vi "Exchange State.vi"(8 "error in (no error)":errorcluster, 9 "Throttle":sgl, 10 "Steering":sgl, 11 "FormulaG API in":refnum<class "FormulaG API.lvclass">) -> (0 "error out":errorcluster, 1 "Paused":bool, 2 "Car State":T1 {"Last Lap" format="%<%M:%S%3u>t"; "Current Lap" format="%<%M:%S%3u>t"}, 3 "FormulaG API out":refnum<class "FormulaG API.lvclass">)   [LabVIEW 2024, in "FormulaG.lvlib" / "FormulaG API.lvclass"]
uses:
  FormulaG API.lvclass
  FormulaG-Common/Car State.ctl
  FormulaG-Common/Ranges.ctl
  FormulaG-Common/Car Info.ctl
  Command.ctl
  FormulaG-Common/Car Control.ctl
  FormulaG API.lvclass/FormulaG API.ctl
  FormulaG-Common/FormulaG-Common.lvlib
  <vilib>/IlluminatedG/IG GodotServer/GodotLV/GodotServer/GodotServer.lvclass
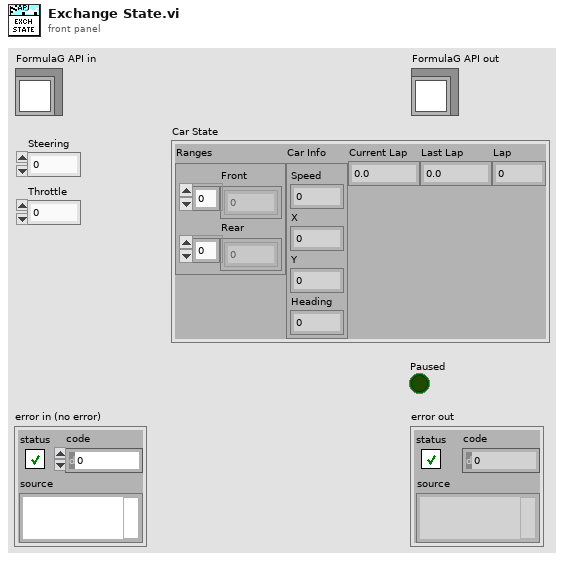
[diagram p1: front panel]
types:
  T1 = typedef "FormulaG-Common.lvlib/Car State.ctl" = cluster{"Ranges":T2, "Car Info":T3, "Current Lap":dbl, "Last Lap":dbl, "Lap":u8}
  T2 = typedef "FormulaG-Common.lvlib/Ranges.ctl" = cluster{"Front":sgl[], "Rear":sgl[]}
  T3 = typedef "FormulaG-Common.lvlib/Car Info.ctl" = cluster{"Speed":sgl, "X":sgl, "Y":sgl, "Heading":sgl}
  T4 = enum16{"big-endian, network order", "native, host order", "little-endian"}
  T5 = typedef "FormulaG-Common.lvlib/Car Control.ctl" = cluster{"Steering (-1 to 1)":sgl, "Throttle (0 to 1)":sgl}
  T6 = cluster{"ID":u8, "Ranges":sgl[], "Info":T3, "Current Lap mS":i64, "Last Lap mS":i64, "Lap":u8, "Paused":u8}
  T7 = typedef "FormulaG.lvlib/FormulaG API.lvclass/Command.ctl" = enum8{"None", "Reset Car", "Request State", "Control Car", "Request Info", "Set Options", "Set Camera", "Set Pause", "Request Time"}
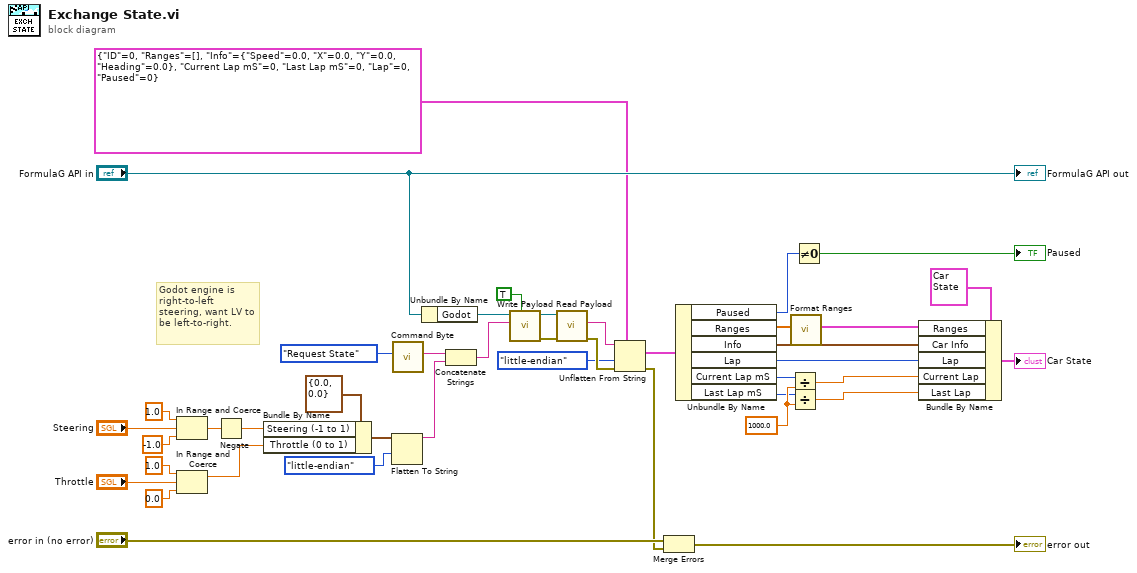
[diagram p0: block diagram]
diagram:
  w27 = 1000.0
  # "Godot engine is right-to-left steering, want LV to be left-to-right."
  n1 = In Range and Coerce(upper limit=sgl 1.0, x="Steering", lower limit=sgl -1.0) -> (coerced(x)=w13:sgl)  [unwired: 1 out]
  n2 = In Range and Coerce(upper limit=sgl 1.0, x="Throttle", lower limit=sgl 0.0) -> (coerced(x)=w8:sgl)  [unwired: 1 out]
  n3 = Negate(x=w13) -> (-x=w16:sgl)
  n4 = Bundle By Name(cluster=T5 {"Steering (-1 to 1)"=0.0, "Throttle (0 to 1)"=0.0} ("Car Control"), "Steering (-1 to 1)"=w16, "Throttle (0 to 1)"=w8) -> (w15:T5)
  n5 = Flatten To String(anything=w15, byte order (0:big-endian, network order)=T4."little-endian") -> (data string=w4:string)  [unwired: 2 in, 2 out]
  n6 = call "Command Byte.vi"("Command"=Command."Request State") -> ("Command Byte"=w34:string)  [unwired: 10 in]
  n7 = Unbundle By Name("FormulaG API in") -> ("Godot"=w35:refnum<class "GodotServer.lvclass">)
  n8 = Concatenate Strings(w34, w4) -> (w5:string)
  n9 = call <vilib>:"Write Payload.vi"("Binary (F = Text)"=TRUE, "Payload"=w5, "GodotServer in"=w35) -> ("error out"=w33:errorcluster, "GodotServer out"=w38:refnum<class "GodotServer.lvclass">)  [unwired: 7 in]
  n10 = call <vilib>:"Read Payload.vi"("error in (no error)"=w33, "GodotServer in"=w38) -> ("error out"=w42:errorcluster, "Payload"=w37:string)  [unwired: 7 in, 1 out]
  n11 = Unflatten From String(type=T6 {"ID"=0, "Ranges"=[], "Info"={"Speed"=0.0, "X"=0.0, "Y"=0.0, "Heading"=0.0}, "Current Lap mS"=0, "Last Lap mS"=0, "Lap"=0, "Paused"=0}, binary string=w37, byte order (0:big-endian, network order)=T4."little-endian", error in (no error)=w42) -> (value=w31:T6, error out=w29:errorcluster)  [unwired: 1 in, 1 out]
  n12 = Merge Errors("error in (no error)", w29) -> (→"error out":errorcluster)
  n13 = Unbundle By Name(w31) -> ("Paused"=w2:u8, "Ranges"=w23:sgl[], "Info"=w21:T3, "Lap"=w3:u8, "Current Lap mS"=w26:i64, "Last Lap mS"=w25:i64)
  n14 = Divide(x=w26, y=w27) -> (x/y=w20:dbl)
  n15 = Divide(x=w25, y=w27) -> (x/y=w19:dbl)
  n16 = call "Format Ranges.vi"("Ranges Array"=w23) -> ("Ranges"=w22:T2)  [unwired: 10 in]
  n17 = Not Equal To 0?(x=w2) -> (x != 0?=→"Paused":bool)
  n18 = Bundle By Name(cluster=T1 {"Ranges"={"Front"=[], "Rear"=[]}, "Car Info"={"Speed"=0.0, "X"=0.0, "Y"=0.0, "Heading"=0.0}, "Current Lap"=0.0, "Last Lap"=0.0, "Lap"=0} ("Car State"), "Ranges"=w22, "Car Info"=w21, "Lap"=w3, "Current Lap"=w20, "Last Lap"=w19) -> (→"Car State":T1)
  "FormulaG API out" <- "FormulaG API in"
